vi "GlobalParcelLocker.vi"() -> ()   [LabVIEW 2017]
panel:
  out "Parcel locker":string
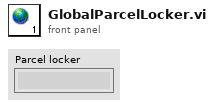
[diagram p1: front panel]
diagram:
